vi "Compile error.vi"(8 "错误输入":errorcluster, 11 "Error":string) -> (3 "Error out":string)   [LabVIEW 2020]
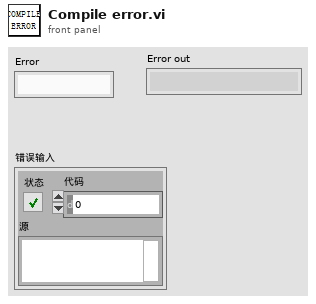
[diagram p1: front panel]
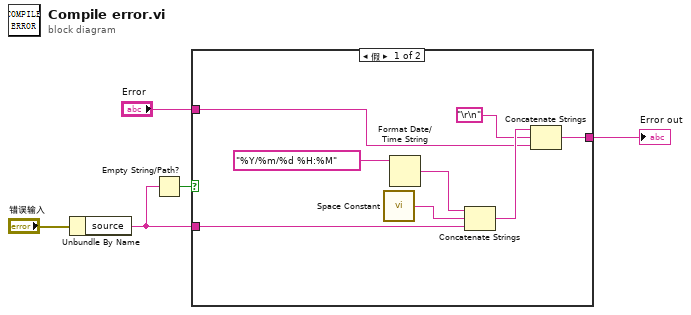
[diagram p0: block diagram]
diagram:
  n1 = Unbundle By Name("错误输入") -> ("source"=w2:string)
  n2 = Empty String/Path?(string/path=w2) -> (empty?=w3:bool)
  n3 = case shown="假" w3 {
    tunnel: [w12 w14] -> w5
    tunnel: w2 -> [w10 _]
    tunnel: "Error" -> [w6 w14]
    frame False {
      n4 = call <vilib>:"Space Constant.vi"() -> ("String"=w9:string)
      n5 = Format Date/Time String(time format string (%c)="%Y/%m/%d %H:%M" ("时间格式字符串(%c)")) -> (date/time string=w7:string)  [unwired: 2 in]
      n6 = Concatenate Strings(w7, w9, w10) -> (w13:string)
      n7 = Concatenate Strings(w13, "\r\n", w6) -> (w12:string)
    }
    frame True {
    }
  }
  "Error out" <- w5
